vi "Set_Hi-Tec_server.vi"(4 "Client Name":string, 6 "Strength (% by volume)":dbl min=0.0 max=5.0 format="%.3f", 7 "Carrier_2 Q (l/min)":dbl=20.0 format="%.2f", 8 "Carrier_1 Q (l/min)":dbl=20.0 format="%.2f", 9 "Mode":enum16{"Control Hi-Tec", "Check Hi-Tec Demands"}(ring)) -> (0 "Flowrates (kg/min)":dbl[](array[numeric]) format="%.2f", 1 "Comment":string)   [LabVIEW 2014]
uses:
  ADAM Client/Sub VIs/ADAM Controls/Ch_description_ADAM.ctl
  ADAM Client/Sub VIs/ADAM Controls/Module_type_ADAM.ctl
  ADAM Client/Sub VIs/ADAM Controls/Function_ADAM.ctl
  ADAM Client/Sub VIs/ADAM Controls/Channel_State.ctl
  ADAM Client/Sub VIs/ADAM Controls/Calib_type_ADAM.ctl
  ADAM Client/Sub VIs/ADAM Controls/Address.ctl
  ADAM Client/Sub VIs/ADAM Controls/Update_scan_value.ctl
  Anemometry/Anemometry Sub Vis/Globals/Gas_management_global.vi
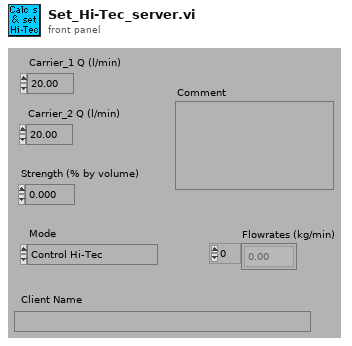
[diagram p1: front panel]
types:
  T1 = enum16{"Append to Global", "Read Global then Clear"}
  T2 = typedef "Calib_type_ADAM.ctl" = enum16{"Raw", "Bx + A", "Cx^2 + Bx + A", "Dx^3 + Cx^2 + Bx + A", "In Band", "Hi-Tec Q", "Hi-Tec M_dot", "Text"}
  T3 = typedef "Module_type_ADAM.ctl" = string
  T4 = typedef "Ch_description_ADAM.ctl" = cluster{"Ch Name":string, "Type":T3, "Function":T5, "Ch State":T6, "Calibration type":T2, "A":dbl, "B":dbl, "C":dbl, "D":dbl, "Comments":string, "Address":T7, "String":string, "Duty":u16}
  T5 = typedef "Function_ADAM.ctl" = enum16{"Analogue Input", "Digital Input", "Event counter", "Event rate", "Analogue Output", "Digital Output", "Relay Output"}
  T6 = typedef "Channel_State.ctl" = enum16{"On", "Off", "Always On", "Always Off"}
  T7 = typedef "Address.ctl" = cluster{"Main":i32, "Ch.":i32, "Sub":i32, "Port Name":string}
  T8 = typedef "Update_scan_value.ctl" = cluster{"Channel Name":string, "New Value":dbl}
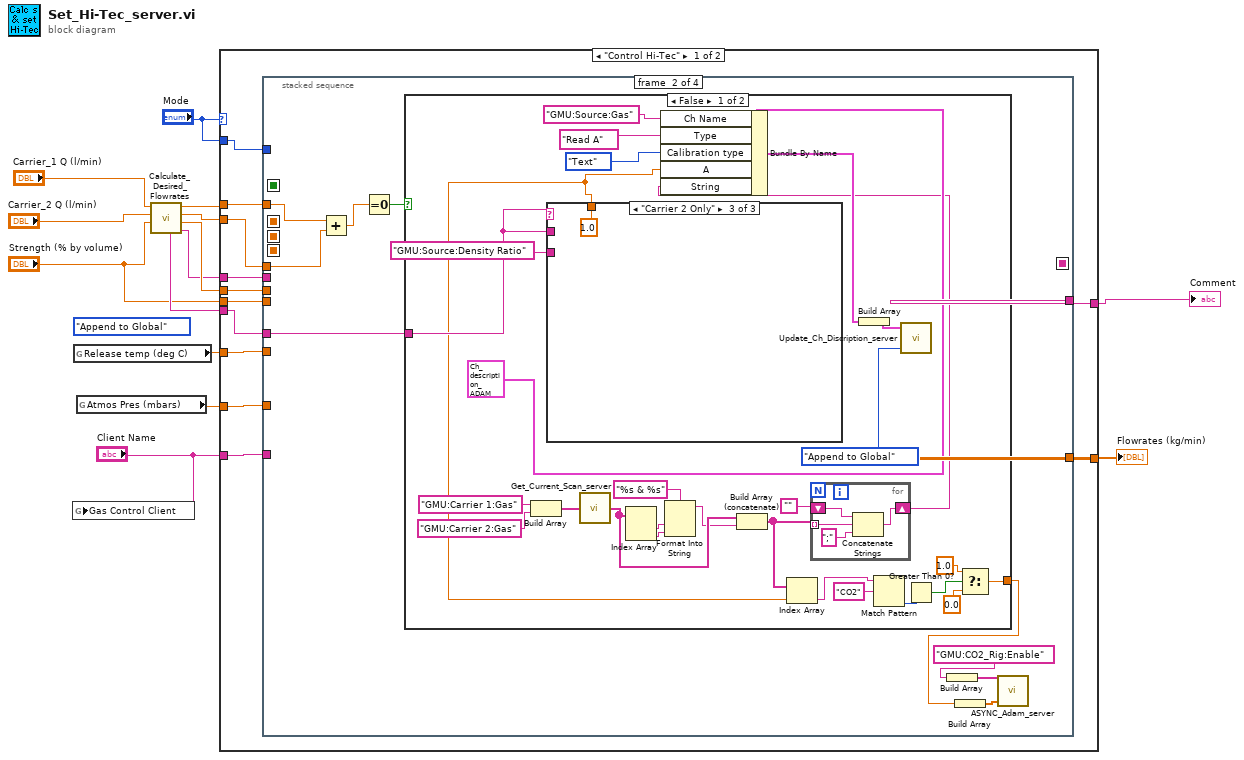
[diagram p0: block diagram]
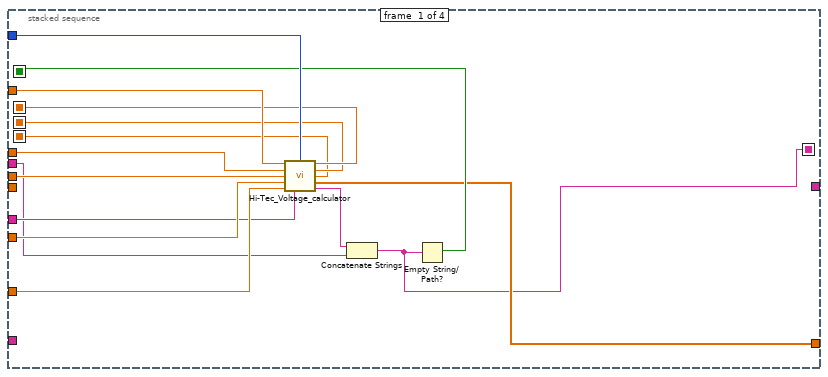
[diagram p2: hidden frame]
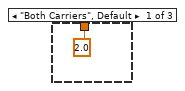
[diagram p3: hidden frame]
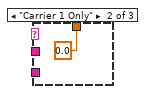
[diagram p4: hidden frame]
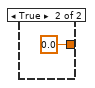
[diagram p5: hidden frame]
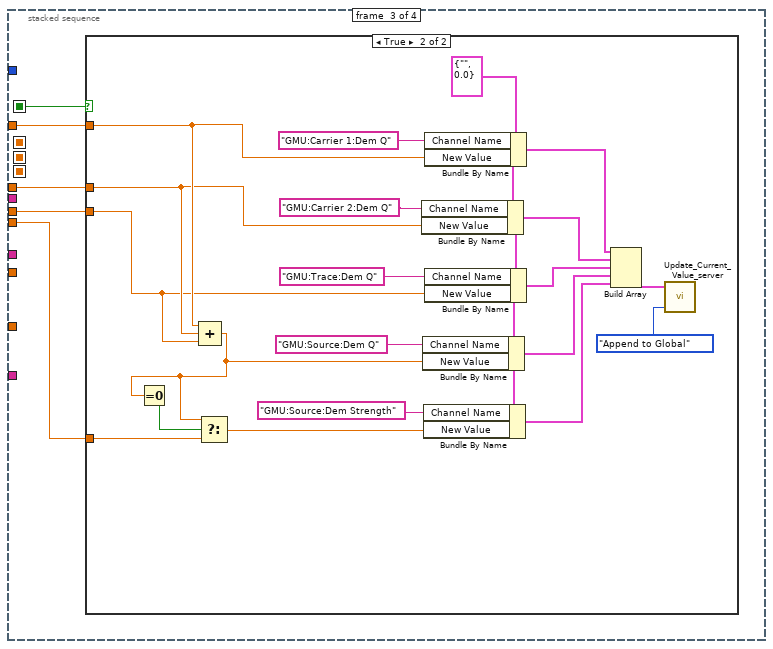
[diagram p6: hidden frame]
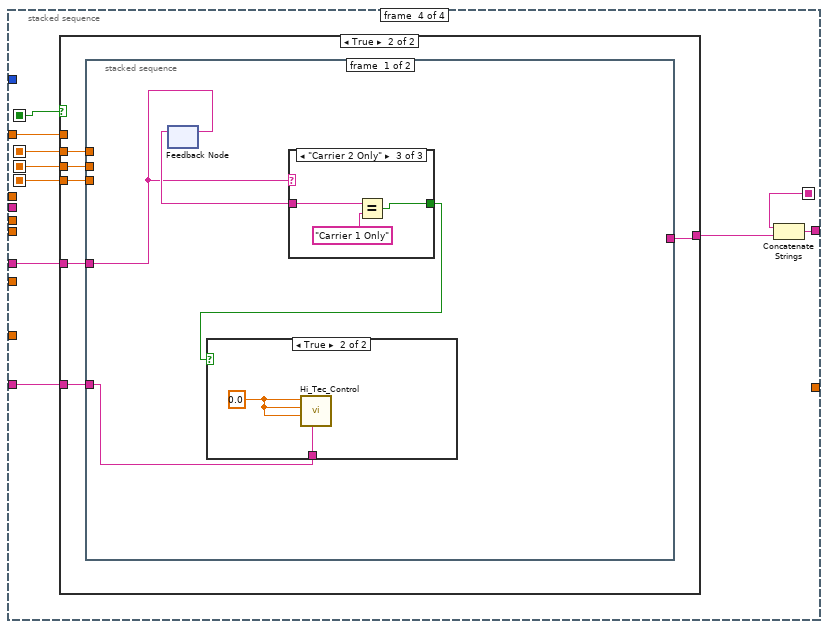
[diagram p8: hidden frame]
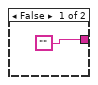
[diagram p9: hidden frame]
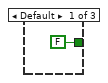
[diagram p10: hidden frame]
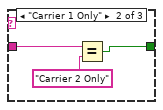
[diagram p11: hidden frame]
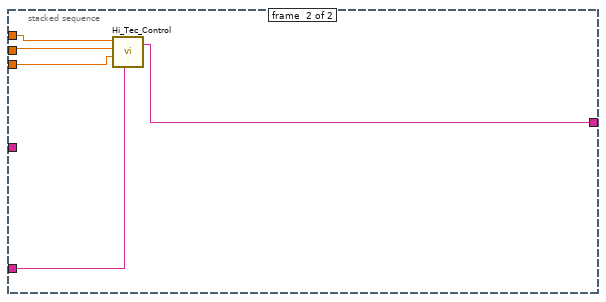
[diagram p13: hidden frame]
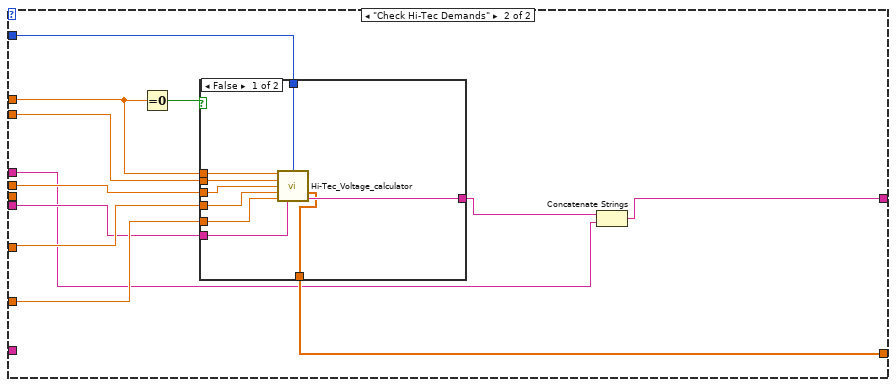
[diagram p14: hidden frame]
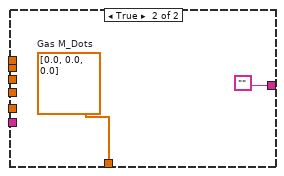
[diagram p15: hidden frame]
diagram:
  (unwired) T1."Append to Global" ("Mode")
  n1 = global write "Gas_management_global.vi" "Gas Control Client"("Client Name") -> ()
  n2 = global read "Gas_management_global.vi" "Release temp (deg C)"() -> (w13:dbl)
  n3 = global read "Gas_management_global.vi" "Atmos Pres (mbars)"() -> (w14:dbl)
  n4 = call "Calculate_Desired_Flowrates.vi"("Strength (% by volume)"="Strength (% by volume)", "Carrier_2 Q (l/min)"="Carrier_2 Q (l/min)", "Carrier_1 Q (l/min)"="Carrier_1 Q (l/min)") -> ("Error Message"=w2:string, "Trace Q l/min"=w5:dbl, "Carrier 2 l/min"=w6:dbl, "Carrier 1 l/min"=w7:dbl, "Carrier Info"=w4:string)  [unwired: 3 in]
  n5 = case shown="\"Control Hi-Tec\"" "Mode" {
    tunnel: w7 -> [w26 w156]
    tunnel: w13 -> [w25 w158]
    tunnel: w14 -> [w24 w157]
    tunnel: [w23 w148] -> w1
    tunnel: [w22 w154] -> w12
    tunnel: "Mode" -> [w21 w153]
    tunnel: "Client Name" -> [w20 _]
    tunnel: w6 -> [w19 w152]
    tunnel: w5 -> [w18 w151]
    tunnel: w4 -> [w17 w150]
    tunnel: "Strength (% by volume)" -> [w16 _]
    tunnel: w2 -> [w15 w147]
    frame "Control Hi-Tec" {
      n6 = stacked-sequence {
        seq-local: [w36 _ _ _] -> [_ _ w91 w117]
        seq-local: [w35 _ _ _] -> [_ _ _ w121]
        seq-local: [w34 _ _ _] -> [_ _ _ w120]
        seq-local: [w33 _ _ _] -> [_ _ _ w119]
        seq-local: [w27 _ _ _] -> [_ _ _ w114]
        tunnel: w19 -> [w39 w42 w89 _]
        tunnel: w26 -> [w38 w43 w90 w116]
        tunnel: w25 -> [w41 _ _ _]
        tunnel: w24 -> [w40 _ _ _]
        tunnel: [_ _ _ w115] -> w23
        tunnel: [w30 _ _ _] -> w22
        tunnel: w21 -> [w37 _ _ _]
        tunnel: w20 -> [_ _ _ w118]
        tunnel: w18 -> [w32 _ w88 _]
        tunnel: w17 -> [w31 w45 _ w112]
        tunnel: w16 -> [_ _ w87 _]
        tunnel: w15 -> [w28 _ _ _]
        frame #0 {
          n7 = call "Hi-Tec_Voltage_calculator.vi"("Carrier_1 Q (l/min)"=w38, "Mode"=w37, "Carrier_2 Q (l/min)"=w39, "Trace Q (l/min)"=w32, "Release temp (deg C)"=w41, "Atmos Pres (mbars)"=w40, "Carrier Info"=w31) -> ("Carrier 1 Voltage"=w35:dbl, "Carrier 2 Voltage"=w34:dbl, "Trace Voltage"=w33:dbl, "Flowrates (kg/min)"=w30:dbl[], "Error Comments"=w29:string)  [unwired: 2 in, 2 out]
          n8 = Concatenate Strings(w29, w28) -> (w27:string)
          n9 = Empty String/Path?(string/path=w27) -> (empty?=w36:bool)
        }
        frame #1 {
          n10 = Add(x=w43, y=w42) -> (x+y=w44:dbl)
          n11 = Equal To 0?(x=w44) -> (x = 0?=w50:bool)
          n12 = case shown="False" w50 {
            tunnel: w45 -> [w76 _]
            tunnel: [w51 0.0 ("f")] -> w46
            frame False {
              n13 = Build Array("GMU:Carrier 1:Gas", "GMU:Carrier 2:Gas") -> (w75:string[])
              n14 = case shown="\"Carrier 2 Only\"" w76 {
                tunnel: "GMU:Source:Density Ratio" -> [_ _ _]
                tunnel: w76 -> [_ _ _]
                tunnel: [2.0 ("A") 0.0 ("A") 1.0 ("A")] -> w58
                frame "Both Carriers", Default {
                }
                frame "Carrier 1 Only" {
                }
                frame "Carrier 2 Only" {
                }
              }
              n15 = call "Get_Current_Scan_server.vi"("Desired Channels"=w75) -> ("String values"=w64:string[])  [unwired: 2 out]
              n16 = Index Array(array=w64) -> (element #1=w67:string, element #2=w66:string)  [unwired: 2 in]
              n17 = Format Into String(format string="%s & %s", w67, w66) -> (resulting string=w63:string)  [unwired: 2 in, 1 out]
              n18 = Build Array (concatenate)(w64, w63) -> (w59:string[])
              n19 = Index Array(array=w59, index=w58) -> (element=w56:string)
              n20 = for {
                shift-right: [w82] -> w60
                shift-left: "" -> [w81]
                tunnel: w59 -> [w80] mode=indexing
                n21 = Concatenate Strings(w81, w80, ";" ("string")) -> (w82:string)
              }
              n22 = Bundle By Name(cluster=T4 {"Ch Name"="", "Type"="", "Function"=enum."Analogue Input", "Ch State"=enum."On", "Calibration type"=enum."Raw", "A"=0.0, "B"=0.0, "C"=0.0, "D"=0.0, "Comments"="", "Address"={"Main"=0, "Ch."=0, "Sub"=0, "Port Name"=""}, "String"="", "Duty"=65535} ("Ch Discription"), "Ch Name"="GMU:Source:Gas", "Type"=T3 "Read A", "Calibration type"=Calib_type_ADAM."Text", "A"=w58, "String"=w60) -> (w69:T4)
              n23 = Build Array(w69) -> (w77:T4[])
              n24 = Match Pattern(string=w56, regular expression="CO2") -> (offset past match=w55:i32)  [unwired: 1 in, 3 out]
              n25 = call "Update_Ch_Discription_server.vi"("Mode"=T1."Append to Global", "Channels to update In"=w77) -> ()  [unwired: 1 in, 1 out]
              n26 = Greater Than 0?(x=w55) -> (x > 0?=w54:bool)
              n27 = Select(t=1.0, s=w54, f=0.0) -> (s? t:f=w51:dbl)
            }
            frame True {
            }
          }
          n28 = Build Array("GMU:CO2_Rig:Enable") -> (w48:string[])
          n29 = Build Array(w46) -> (w49:dbl[])
          n30 = call "ASYNC_Adam_server.vi"("Values"=w49, "Channel Names"=w48) -> ()  [unwired: 1 in, 3 out]
        }
        frame #2 {
          n31 = case shown="True" w91 {
            tunnel: w90 -> [_ w102]
            tunnel: w89 -> [_ w101]
            tunnel: w88 -> [_ w100]
            tunnel: w87 -> [_ w98]
            frame False {
            }
            frame True {
              w97 = T8 {"Channel Name"="", "New Value"=0.0} ("Update Scan Value Cluster")
              n32 = Compound Arithmetic op=ADD(w102, w101, w100) -> (w99:dbl)
              n33 = Equal To 0?(x=w99) -> (x = 0?=w107:bool)
              n34 = Select(t=w99, s=w107, f=w98) -> (s? t:f=w106:dbl)
              n35 = Bundle By Name(cluster=w97, "Channel Name"="GMU:Carrier 2:Dem Q", "New Value"=w101) -> (w95:T8)
              n36 = Bundle By Name(cluster=w97, "Channel Name"="GMU:Source:Dem Q", "New Value"=w99) -> (w93:T8)
              n37 = Bundle By Name(cluster=w97, "Channel Name"="GMU:Source:Dem Strength", "New Value"=w106) -> (w92:T8)
              n38 = Bundle By Name(cluster=w97, "Channel Name"="GMU:Carrier 1:Dem Q", "New Value"=w102) -> (w96:T8)
              n39 = Bundle By Name(cluster=w97, "Channel Name"="GMU:Trace:Dem Q", "New Value"=w100) -> (w94:T8)
              n40 = Build Array(w96, w95, w94, w93, w92) -> (w109:T8[])
              n41 = call "Update_Current_Value_server.vi"("Mode"=T1."Append to Global", "Update array in"=w109) -> ()  [unwired: 1 in, 1 out]
            }
          }
        }
        frame #3 {
          n42 = case shown="True" w117 {
            tunnel: w121 -> [_ w128]
            tunnel: w120 -> [_ w127]
            tunnel: w119 -> [_ w126]
            tunnel: w118 -> [_ w125]
            tunnel: w116 -> [_ _]
            tunnel: ["" w124] -> w113
            tunnel: w112 -> [_ w123]
            frame False {
            }
            frame True {
              n43 = stacked-sequence {
                tunnel: w128 -> [_ w146]
                tunnel: w127 -> [_ w145]
                tunnel: w126 -> [_ w144]
                tunnel: w125 -> [w132 w143]
                tunnel: [_ w142] -> w124
                tunnel: w123 -> [w129 _]
                frame #0 {
                  n44 = feedback-in #1(w129) -> ()
                  n45 = feedback #1() -> (w131:string)  [unwired: 1 in]
                  n46 = case shown="\"Carrier 2 Only\"" w129 {
                    tunnel: w131 -> [_ w136 w139]
                    tunnel: [FALSE w134 w137] -> w130
                    frame Default {
                    }
                    frame "Carrier 1 Only" {
                      n47 = Equal?(x=w136, y="Carrier 2 Only") -> (x = y?=w134:bool)
                    }
                    frame "Carrier 2 Only" {
                      n48 = Equal?(x=w139, y="Carrier 1 Only") -> (x = y?=w137:bool)
                    }
                  }
                  n49 = case shown="True" w130 {
                    tunnel: w132 -> [_ w141]
                    frame False {
                    }
                    frame True {
                      w140 = 0.0 ("Carrier 1 Voltage")
                      n50 = call "Hi_Tec_Control.vi"("Carrier 1 Voltage"=w140, "Carrier 2 Voltage"=w140, "Trace Voltage"=w140, "Client Name"=w141) -> ()  [unwired: 3 out]
                    }
                  }
                }
                frame #1 {
                  n51 = call "Hi_Tec_Control.vi"("Carrier 1 Voltage"=w146, "Carrier 2 Voltage"=w145, "Trace Voltage"=w144, "Client Name"=w143) -> ("Scan Comments"=w142:string)  [unwired: 2 out]
                }
              }
            }
          }
          n52 = Concatenate Strings(w114, w113) -> (w115:string)
        }
      }
    }
    frame "Check Hi-Tec Demands" {
      n53 = Equal To 0?(x=w156) -> (x = 0?=w155:bool)
      n54 = case shown="False" w155 {
        tunnel: w152 -> [w167 _]
        tunnel: w158 -> [w166 _]
        tunnel: w157 -> [w165 _]
        tunnel: [w164 ""] -> w149
        tunnel: w156 -> [w163 _]
        tunnel: [w160 w168] -> w154
        tunnel: w153 -> [w162 _]
        tunnel: w151 -> [w161 _]
        tunnel: w150 -> [w159 _]
        frame False {
          n55 = call "Hi-Tec_Voltage_calculator.vi"("Carrier_1 Q (l/min)"=w163, "Mode"=w162, "Carrier_2 Q (l/min)"=w167, "Trace Q (l/min)"=w161, "Release temp (deg C)"=w166, "Atmos Pres (mbars)"=w165, "Carrier Info"=w159) -> ("Flowrates (kg/min)"=w160:dbl[], "Error Comments"=w164:string)  [unwired: 1 in, 6 out]
        }
        frame True {
          w168 = dbl[] [0.0, 0.0, 0.0]  # Gas M_Dots
        }
      }
      n56 = Concatenate Strings(w149, w147) -> (w148:string)
    }
  }
  "Comment" <- w1
  "Flowrates (kg/min)" <- w12
